vi "String.String to Number Conversion and Check.vi"(11 "String":string) -> (2 "IsNum":bool, 3 "Numeric":dbl)   [LabVIEW 2019]
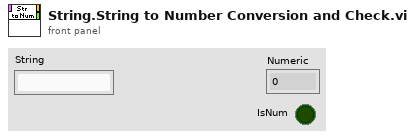
[diagram p1: front panel]
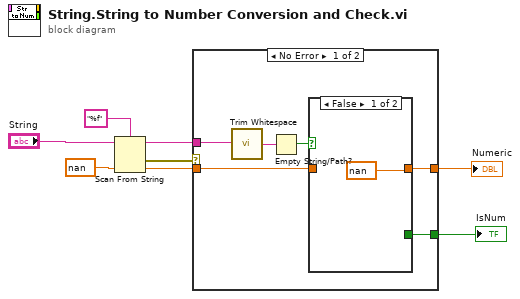
[diagram p0: block diagram]
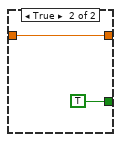
[diagram p2: hidden frame]
diagram:
  n1 = Scan From String(format string="%f", input string="String", default 1=nan ("input 1")) -> (remaining string=w1:string, error out=w4:errorcluster, output 1=w5:dbl)  [unwired: 2 in, 1 out]
  n2 = case shown="No Error" w4 {
    tunnel: w5 -> [w11 w18]
    tunnel: [w10 w18] -> w3
    tunnel: [w9 _] -> w2
    tunnel: w1 -> [w14 _]
    frame No Error {
      n3 = call <vilib>:"Trim Whitespace.vi"("string"=w14) -> ("trimmed string"=w13:string)  [unwired: 1 in]
      n4 = Empty String/Path?(string/path=w13) -> (empty?=w12:bool)
      n5 = case shown="False" w12 {
        tunnel: w11 -> [_ w17]
        tunnel: [nan ("input 1") w17] -> w10
        tunnel: [_ TRUE] -> w9
        frame False {
        }
        frame True {
        }
      }
    }
    frame Error {
    }
  }
  "Numeric" <- w3
  "IsNum" <- w2
